vi "GUI_BELLA-shotcontrol.vi"() -> ()   [LabVIEW 2013]
uses:
  shared programs/GUI_Template/GUI_master/tcp_new_data_event.ctl
  shared programs/GUI_Template/GUI_master/tcp new data cluster.ctl
panel:
  in  "Mode::1":enum16{"Continuous", "Single Shot"}(ring)
  in  "fire::1":string
  in  "RepRate::1":dbl=0.001 caption="RepRate" min=0.1 max=10.0 format="%_4p"
  in  "GUIdevice 1":string="BELLA-shotcontrol"
  in  "insert tag":bool=TRUE
  in  "stop":bool
  out "tcp data event":T1
  out "error IO 2":errorcluster
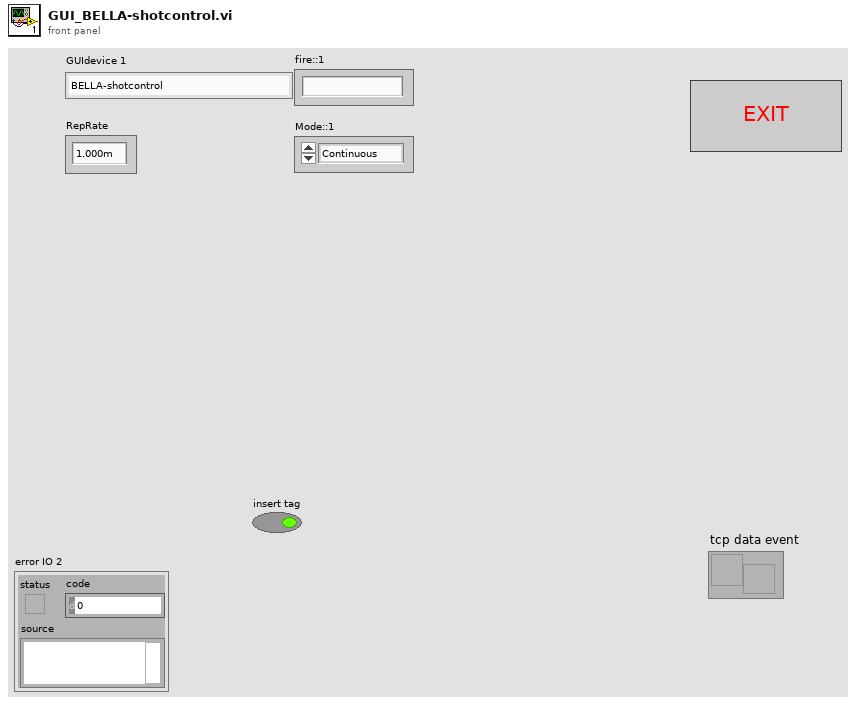
[diagram p1: front panel]
types:
  T1 = typedef "tcp_new_data_event.ctl" = refnum<user-event>
  T2 = typedef "tcp new data cluster.ctl" = cluster{"EventEnum":enum16{"new data", "connection status update"}, "Device name":string}
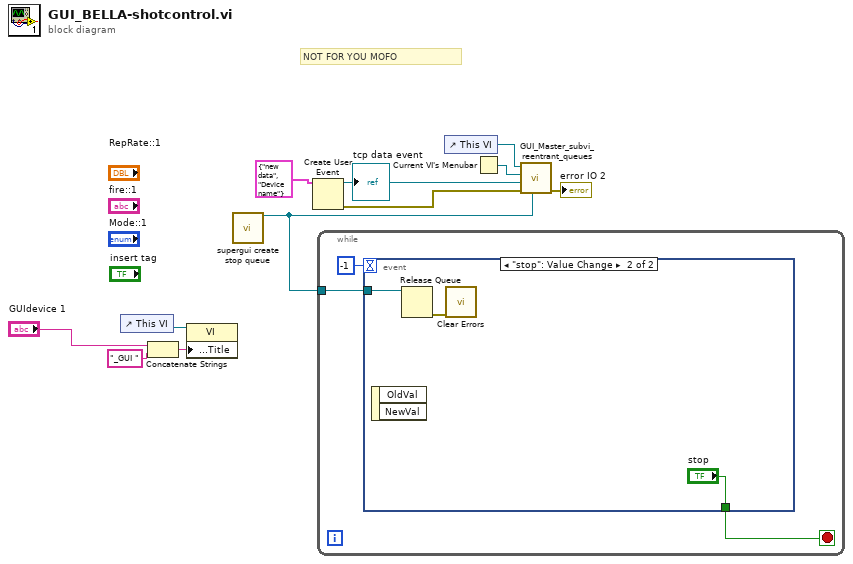
[diagram p0: block diagram]
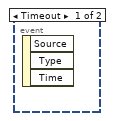
[diagram p2: hidden frame]
diagram:
  # "NOT FOR YOU MOFO"
  n1 = control-ref of="This VI"() -> (w4:refnum<vi>)
  n2 = Concatenate Strings("GUIdevice 1", "_GUI ") -> (w3:string)
  n3 = property class="VI"(reference=w4, "Front Panel.Title"=w3) -> ()  [unwired: 1 in, 2 out]
  n4 = call "supergui create stop queue.vi"() -> ("STOP Queue out"=w5:refnum<queue>)  [unwired: 11 in]
  n5 = Create User Event(user event datatype=T2 {"EventEnum"=enum."new data", "Device name"="Device name"} ("New Event")) -> (user event=w6:refnum<user-event>, error out=w7:errorcluster)  [unwired: 1 in]
  "tcp data event" <- w6
  n6 = while {
    tunnel: w5 -> [w12]
    stop <- w13 stop-if-true
    n7 = event shown="[1] \"stop\": Value Change" {
      selector: _ -> [_ _]
      dyn-events: _ -> [_ _]
      timeout: -1 -> [_ _]
      tunnel: [_ "stop"] -> w13
      tunnel: w12 -> [_ w16]
      event Timeout {
        n8 = event-data() -> ()  [unwired: 1 in, 3 out]
      }
      event "stop": Value Change {
        n9 = event-data() -> ()  [unwired: 1 in, 2 out]
        n10 = Release Queue(queue=w16) -> (error out=w15:errorcluster)  [unwired: 2 in, 2 out]
        n11 = call <vilib>:"Clear Errors.vi"("error in (no error)"=w15) -> ()  [unwired: 6 in, 1 out]
      }
    }
  }
  n12 = control-ref of="This VI"() -> (w10:refnum<vi>)
  n13 = Current VI's Menubar() -> (w9:refnum<k9>)
  n14 = call "GUI_Master_subvi_reentrant_queues.vi"("STOP Queue in"=w5, "error in (no error)"=w7, "tcp data event"=w6, "Caller menu reference"=w9, "Caller VI ref"=w10) -> ("error out"=→"error IO 2":errorcluster)  [unwired: 6 in]
